vi "UpdateOverlay.vi"(7 "ROI Entry":T9 {"Analysis_Setting"."Analysis_Type" items=["None", "PatternMatch", "Edge Detection", "Barcode 1D", "Barcode 2D", "Clamp", "Clamp MAX", "Particle", "Histogram", "Straight Edge", "Circle", "Shape Detect", "OCR", "Contour", "ColorMatch"]}, 8 "error in (no error)":errorcluster, 10 "AnalysisResult":variant) -> (0 "error out":errorcluster)   [LabVIEW 2019]
uses:
  [Global] Image.vi
  [Global] Analyze Image.vi
  Analysis/Controls/Analysis_Type.ctl
  Process/Controls/Process_Type.ctl
  Process/Controls/Process_Setting.ctl
  Analysis/Controls/Analysis_Setting.ctl
  Controls/Vision_DataEntry.ctl
  <vilib>/vision/Measure.llb/Edge New.ctl
panel:
  in  "Straight Edge Cluster Array":T1(array[cluster])
  in  "Clamp output cluster":T2
  in  "Particle output cluster":T3
  in  "Clamp MAX output cluster":T4
  in  "Barcode 1D output cluster":T5
  in  "Edge Detectionoutput cluster":T7 {"?"."Edge Information"."Distance (Real-World)" format="%.2f"; "?"."Edge Information"."Location (Real-World)"."Y" format="%.2g"; "?"."Edge Information"."Location (Real-World)"."X" format="%.2f"; "?"."Edge Information"."Noise" format="%.2f"; "?"."Edge Information"."Location (Pixel)"."Y" format="%.2g"; "?"."Edge Information"."Location (Pixel)"."X" format="%.2f"; "?"."Edge Information"."Strength" format="%.2f"; "?"."Edge Information"."Distance (Pixel)" format="%.2f"}
  in  "Barcode 2D output cluster":T8
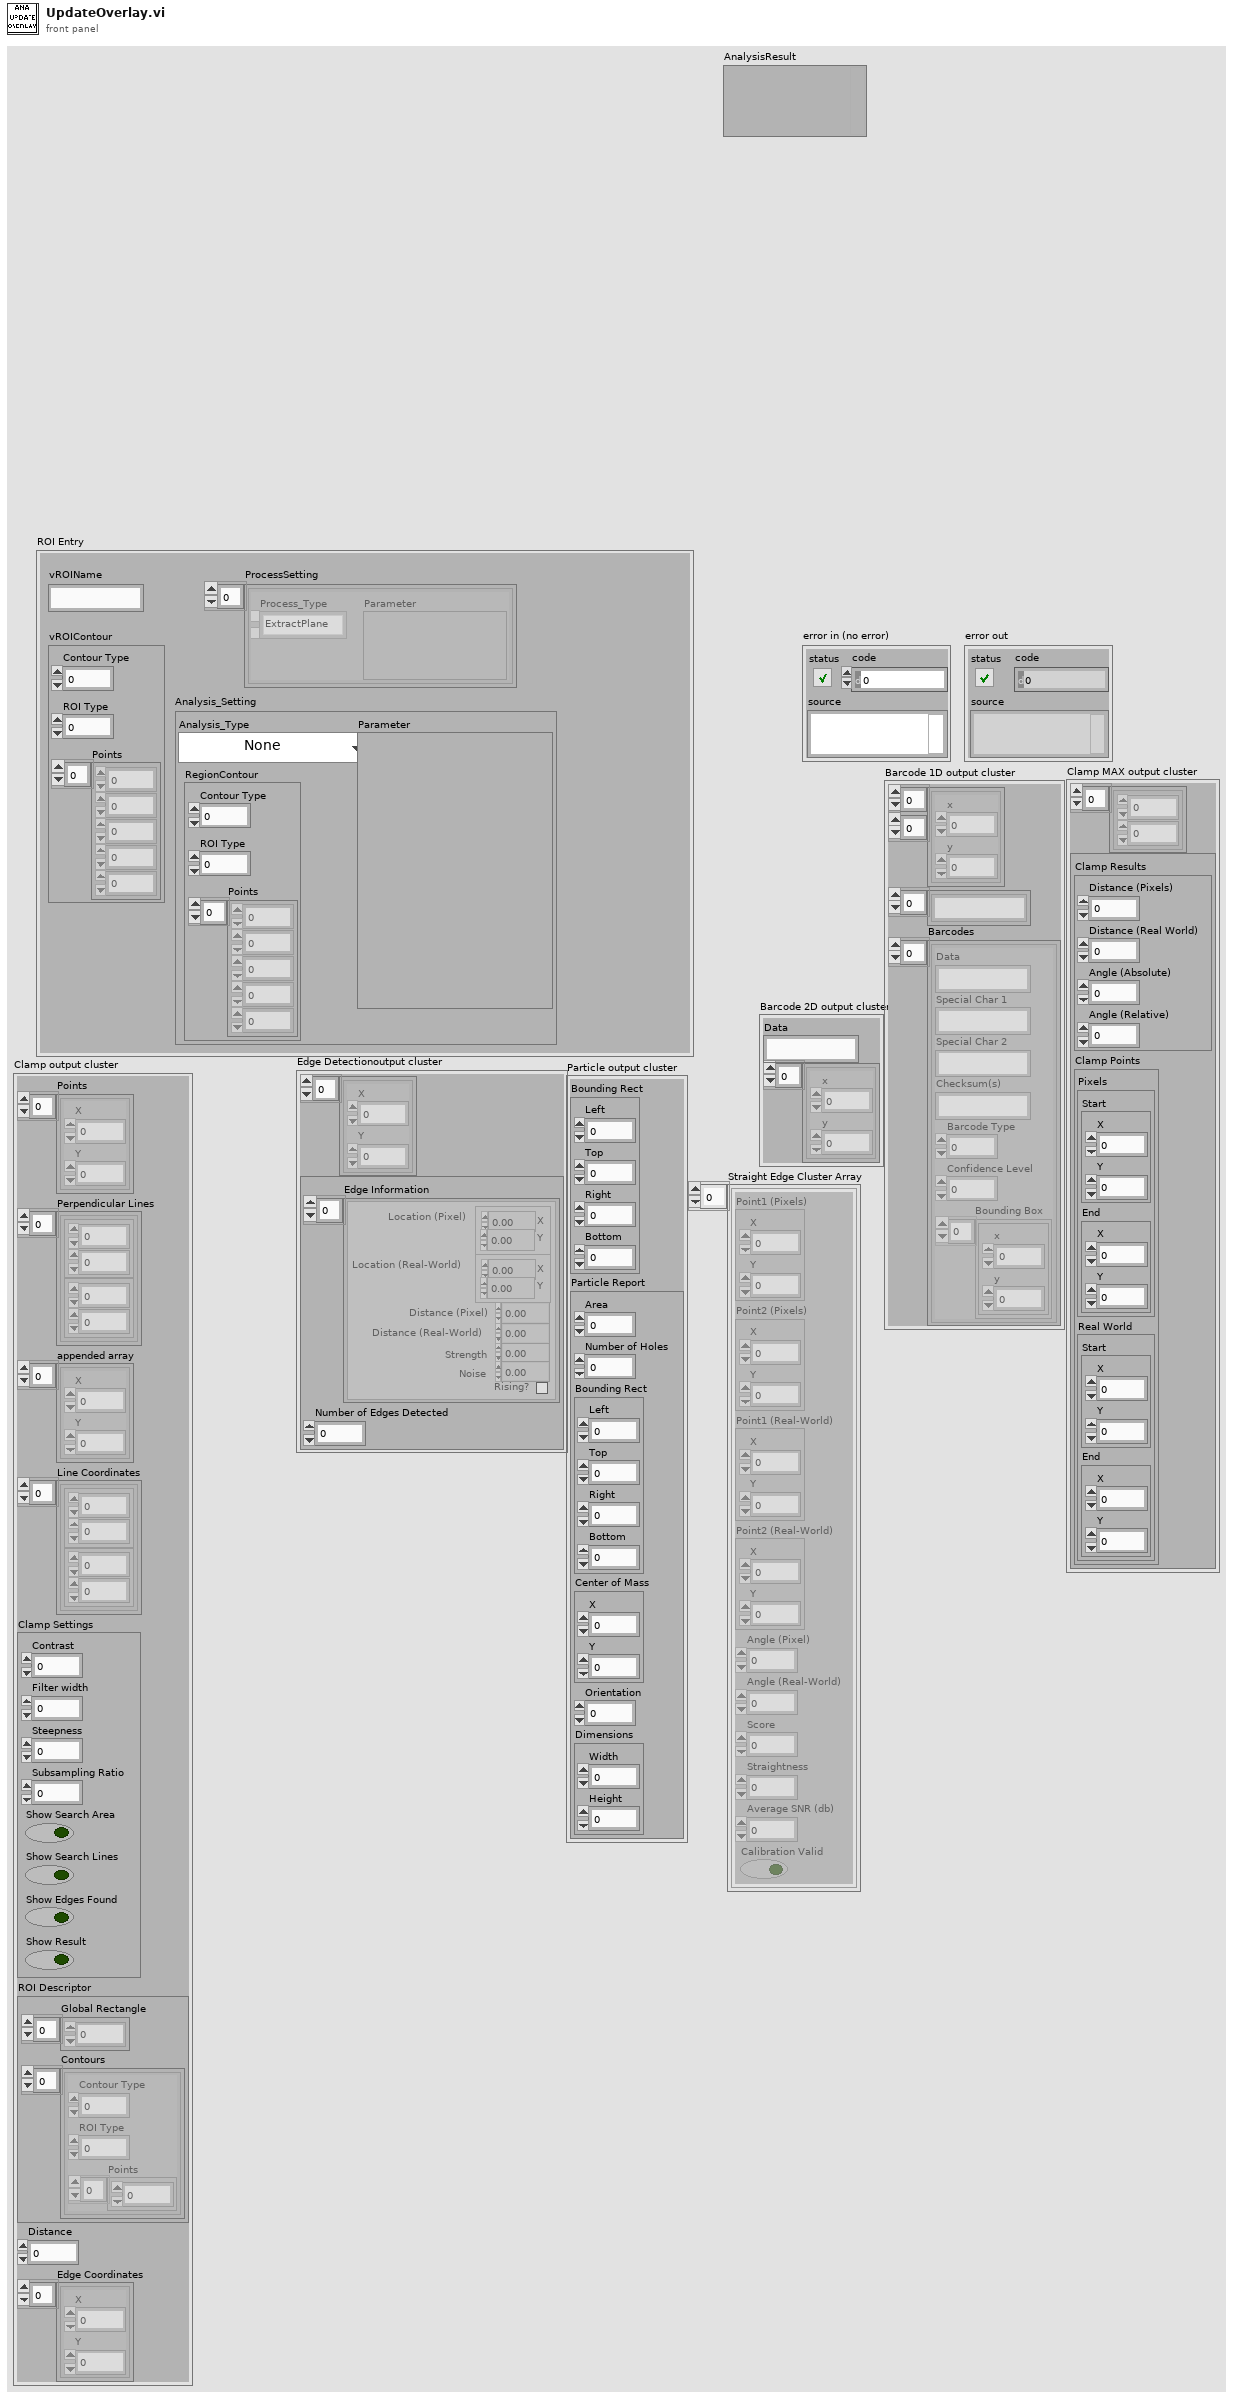
[diagram p1: front panel]
types:
  T1 = cluster{"Point1 (Pixels)":cluster{"X":sgl, "Y":sgl}, "Point2 (Pixels)":cluster{"X":sgl, "Y":sgl}, "Point1 (Real-World)":cluster{"X":sgl, "Y":sgl}, "Point2 (Real-World)":cluster{"X":sgl, "Y":sgl}, "Angle (Pixel)":dbl, "Angle (Real-World)":dbl, "Score":dbl, "Straightness":dbl, "Average SNR (db)":dbl, "Calibration Valid":bool}[]
  T2 = cluster{"Points":cluster{"X":sgl, "Y":sgl}[], "Perpendicular Lines":cluster{cluster{sgl, sgl}, cluster{sgl, sgl}}[], "appended array":cluster{"X":sgl, "Y":sgl}[], "Line Coordinates":cluster{cluster{sgl, sgl}, cluster{sgl, sgl}}[], "Clamp Settings":cluster{"Contrast":i32, "Filter width":i32, "Steepness":i32, "Subsampling Ratio":u32, "Show Search Area":bool, "Show Search Lines":bool, "Show Edges Found":bool, "Show Result":bool}, "ROI Descriptor":cluster{"Global Rectangle":i32[], "Contours":cluster{"Contour Type":u32, "ROI Type":u32, "Points":i32[]}[]}, "Distance":sgl, "Edge Coordinates":cluster{"X":sgl, "Y":sgl}[]}
  T3 = cluster{"Bounding Rect":cluster{"Left":dbl, "Top":dbl, "Right":dbl, "Bottom":dbl}, "Particle Report":cluster{"Area":dbl, "Number of Holes":dbl, "Bounding Rect":cluster{"Left":dbl, "Top":dbl, "Right":dbl, "Bottom":dbl}, "Center of Mass":cluster{"X":dbl, "Y":dbl}, "Orientation":dbl, "Dimensions":cluster{"Width":dbl, "Height":dbl}}}
  T4 = cluster{cluster{dbl, dbl}[], cluster{"Clamp Results":cluster{"Distance (Pixels)":dbl, "Distance (Real World)":dbl, "Angle (Absolute)":dbl, "Angle (Relative)":dbl}, "Clamp Points":cluster{"Pixels ":cluster{"Start":cluster{"X":dbl, "Y":dbl}, "End":cluster{"X":dbl, "Y":dbl}}, "Real World":cluster{"Start":cluster{"X":dbl, "Y":dbl}, "End":cluster{"X":dbl, "Y":dbl}}}}}
  T5 = cluster{cluster{"x":sgl, "y":sgl}[][], string[], "Barcodes":cluster{"Data":string, "Special Char 1":string, "Special Char 2":string, "Checksum(s)":string, "Barcode Type":u32, "Confidence Level":sgl, "Bounding Box":cluster{"x":sgl, "y":sgl}[]}[]}
  T6 = typedef "Edge New.ctl" = cluster{"Location (Pixel)":cluster{"X":sgl, "Y":sgl}, "Location (Real-World)":cluster{"X":sgl, "Y":sgl}, "Distance (Pixel)":dbl, "Distance (Real-World)":dbl, "Strength":dbl, "Noise":dbl, "Rising?":bool}
  T7 = cluster{cluster{"X":sgl, "Y":sgl}[], cluster{"Edge Information":T6[], "Number of Edges Detected":i32}}
  T8 = cluster{"Data":string, cluster{"x":sgl, "y":sgl}[]}
  T9 = typedef "Vision_DataEntry.ctl" = cluster{"vROIName":string, "vROIContour":cluster{"Contour Type":u32, "ROI Type":u32, "Points":i32[]}, "ProcessSetting":T10[], "Analysis_Setting":T12}
  T10 = typedef "Process_Setting.ctl" = cluster{"Process_Type":T11, "Parameter":variant}
  T11 = typedef "Process_Type.ctl" = enum16{"None", "ExtractPlane", "BinaryMono", "Operators", "GrayMorphology", "Filters", "Lookup Table", "Particle Filter", "Mask"}
  T12 = typedef "Analysis_Setting.ctl" = cluster{"Analysis_Type":T13, "RegionContour":cluster{"Contour Type":u32, "ROI Type":u32, "Points":i32[]}, "Parameter":variant}
  T13 = typedef "Analysis_Type.ctl" = u16
  T14 = typedef "IMAQ Image.ctl" = refnum<image>
  T15 = typedef "ROI Descriptor" = cluster{"Global Rectangle":i32[], "Contours":cluster{"ID":enum32{"External", "Internal"}, "Type":u32, "Coordinates":i32[]}[]}
  T16 = cluster{"ROI Descriptor out":T15, cluster{sgl, sgl}, "Angle":sgl, "Score":sgl}[]
  T17 = typedef "IMAQ Rectangle" = cluster{"Left":i32, "Top":i32, "Right":i32, "Bottom":i32, "Rotation":dbl}
  T18 = typedef "IMAQ Point" = cluster{"X":sgl, "Y":sgl}
  T19 = cluster{"Contrast":i32, "Filter width":i32, "Steepness":i32, "Subsampling Ratio":u32, "Show Search Area":bool, "Show Search Lines":bool, "Show Edges Found":bool, "Show Result":bool}
  T20 = cluster{"Global Rectangle":i32[], "Contours":cluster{"Contour Type":u32, "ROI Type":u32, "Points":i32[]}[]}
  T21 = cluster{"Left":dbl, "Top":dbl, "Right":dbl, "Bottom":dbl}
  T22 = cluster{"ROI Descriptor out":cluster{"Global Rectangle":i32[], "Contours":cluster{"ID":enum32{"External", "Internal"}, "Type":u32, "Coordinates":i32[]}[]}, "Output value":dbl}
  T23 = cluster{"Global Rectangle":i32[], "Contours":cluster{"ID":enum32{"External", "Internal"}, "Type":u32, "Coordinates":i32[]}[]}
  T24 = cluster{"ID":enum32{"External", "Internal"}, "Type":u32, "Coordinates":i32[]}[]
  T25 = cluster{"ID":enum32{"External", "Internal"}, "Type":u32, "Coordinates":i32[]}
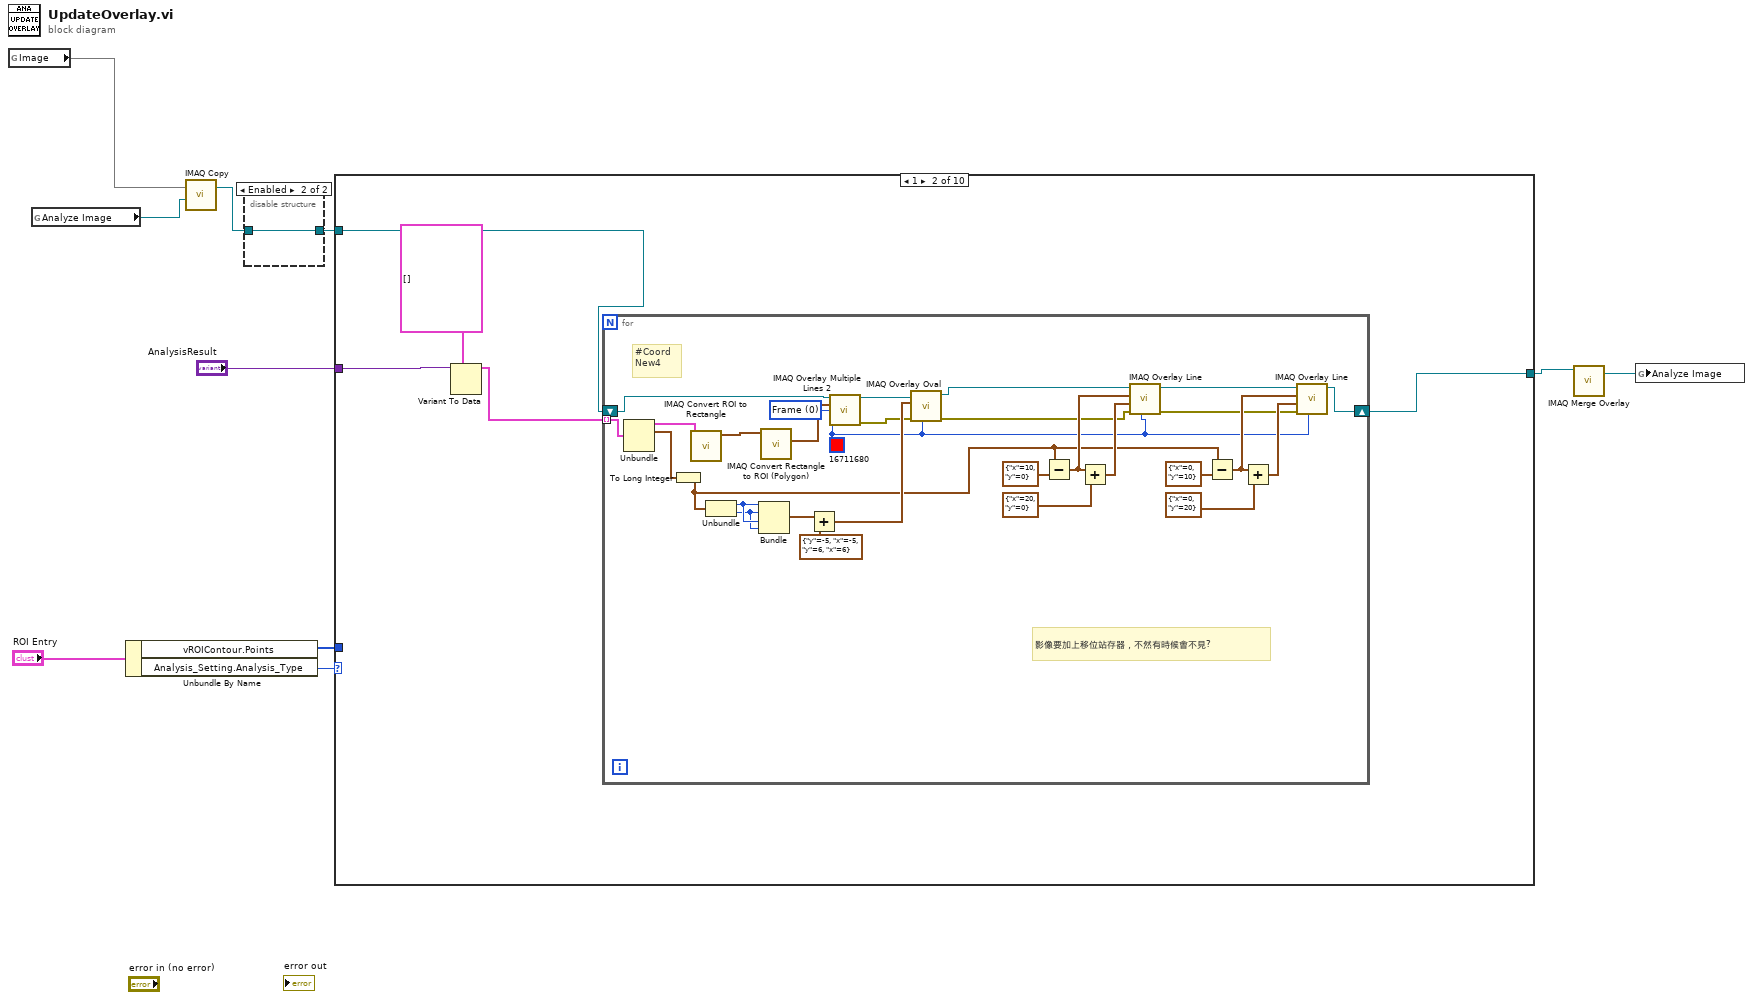
[diagram p0: block diagram]
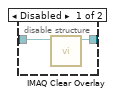
[diagram p2: hidden frame]
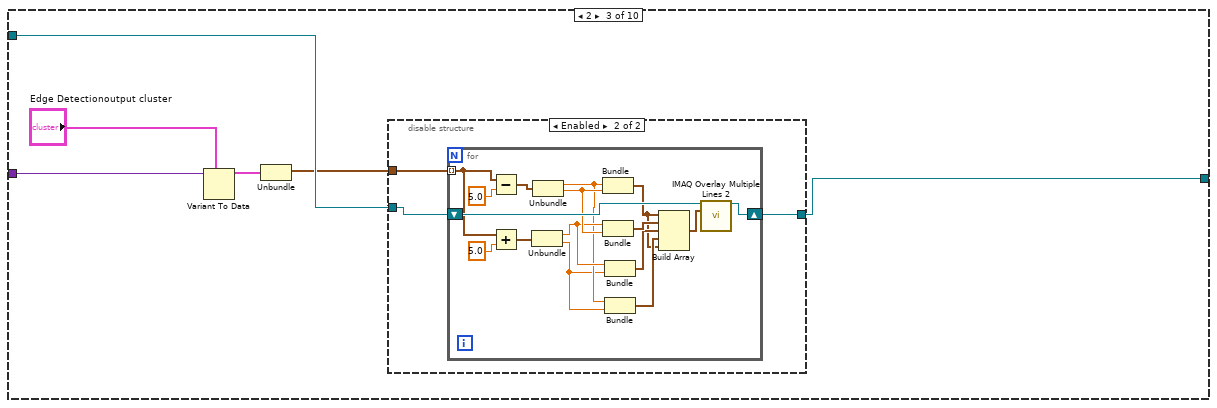
[diagram p4: hidden frame]
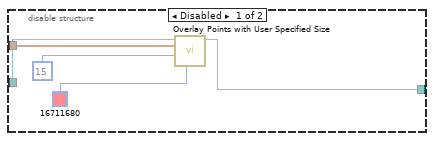
[diagram p5: hidden frame]
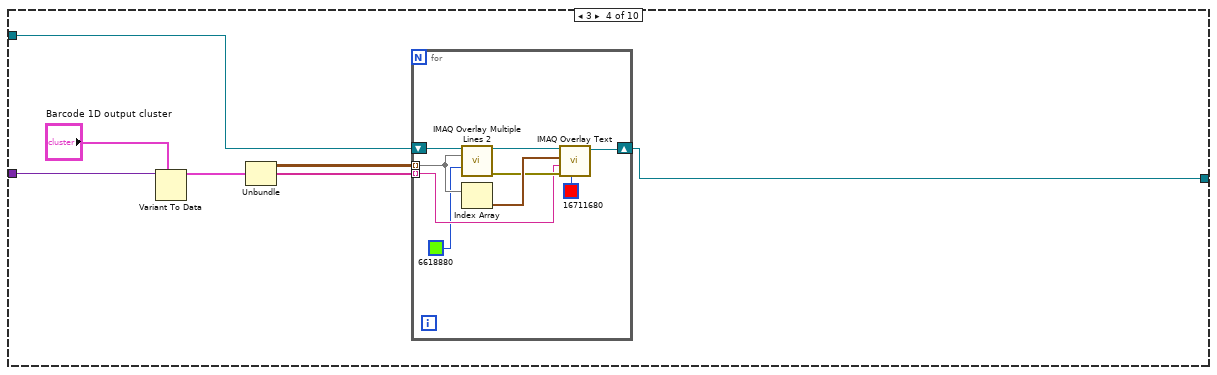
[diagram p6: hidden frame]
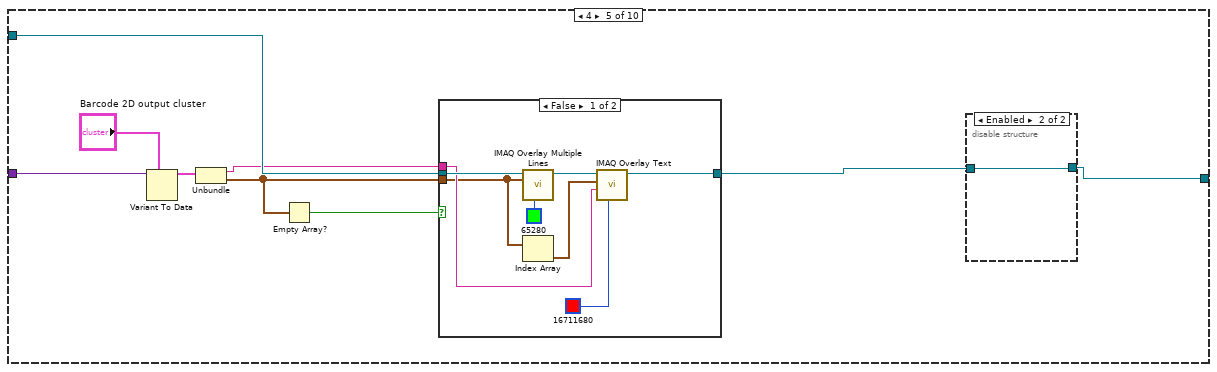
[diagram p7: hidden frame]
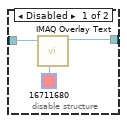
[diagram p9: hidden frame]
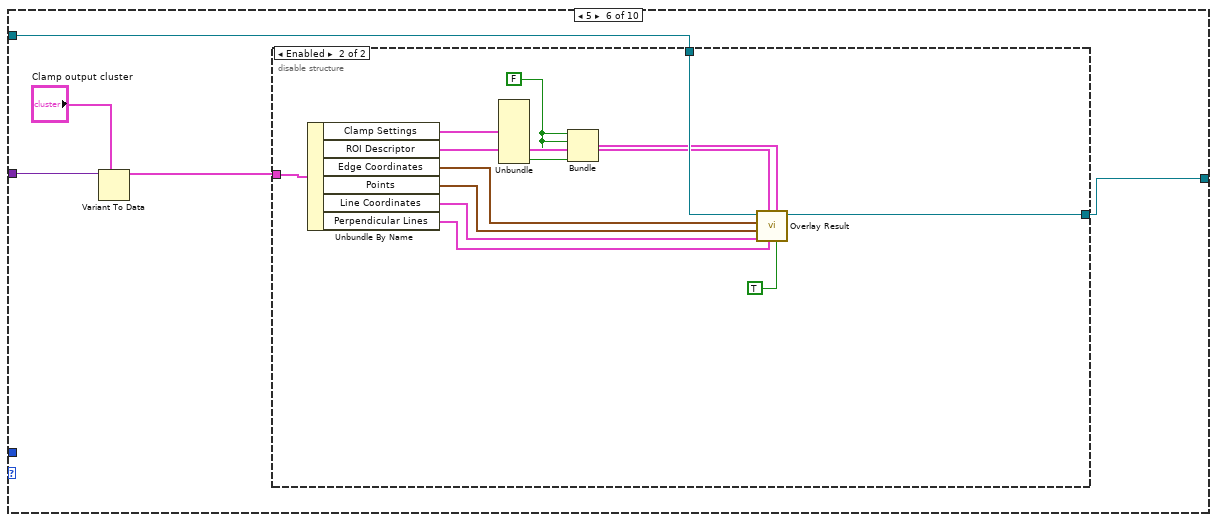
[diagram p10: hidden frame]
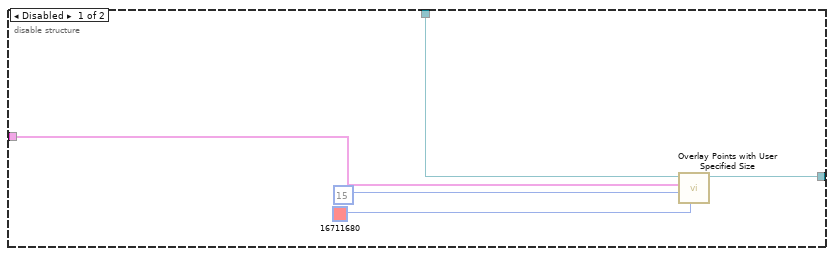
[diagram p11: hidden frame]
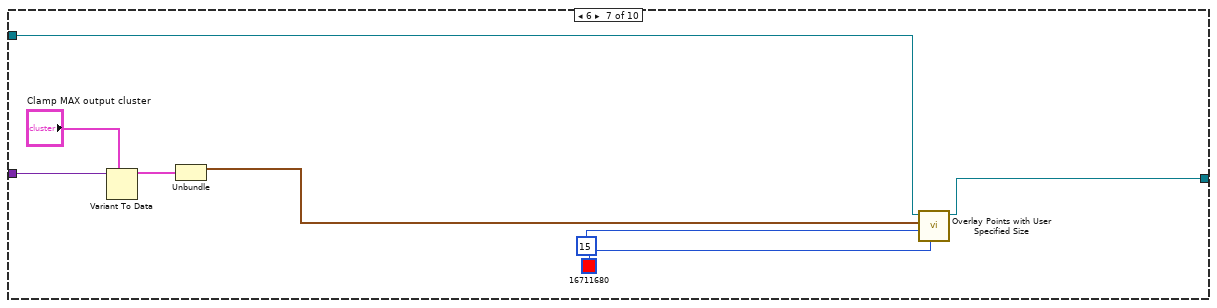
[diagram p12: hidden frame]
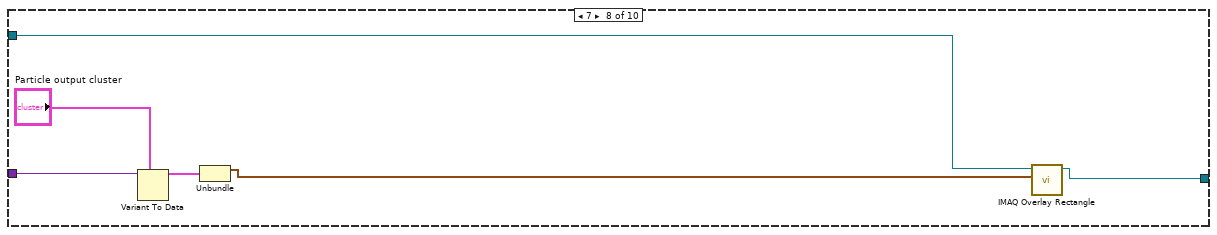
[diagram p13: hidden frame]
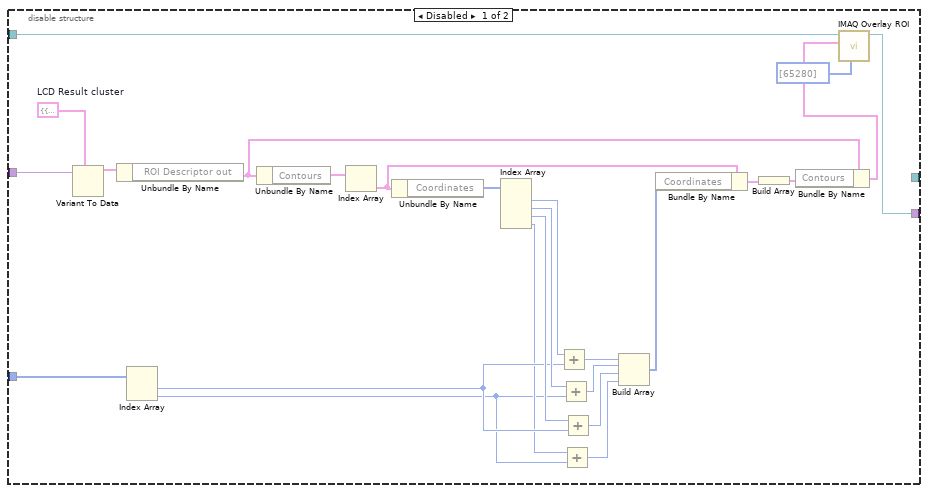
[diagram p15: hidden frame]
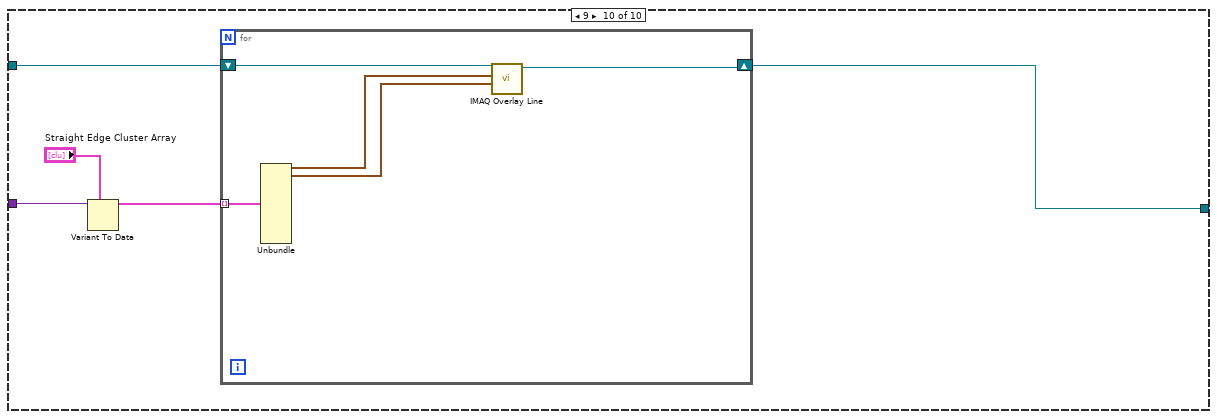
[diagram p16: hidden frame]
diagram:
  n1 = global read "[Global] Image.vi" "Image"() -> (w5)
  n2 = global read "[Global] Analyze Image.vi" "Analyze Image"() -> (w4:T14)
  n3 = Unbundle By Name("ROI Entry") -> ("vROIContour.Points"=w8:i32[], "Analysis_Setting.Analysis_Type"=w7:T13)
  n4 = call "IMAQ Copy"("Image Dst"=w4, "Image Src"=w5) -> ("Image Dst Out"=w3:T14)  [unwired: 4 in, 1 out]
  n5 = disable-structure shown="Enabled" {
    disable-tunnel: w3 -> [w12 w13]
    disable-tunnel: [w11 w13] -> w10
    frame Disabled {
      n6 = call "IMAQ Clear Overlay"("Image"=w12) -> ("Image Out"=w11:T14)  [unwired: 9 in, 1 out]
    }
    frame Enabled {
    }
  }
  n7 = case shown="1" w7 {
    tunnel: "AnalysisResult" -> [_ w19 w54 w85 w103 w121 w147 w153 w157 w189]
    tunnel: w8 -> [_ _ _ _ _ _ _ _ w155 _]
    tunnel: w10 -> [w14 w18 w53 w81 w100 w120 w144 w152 w156 w186]
    tunnel: [w14 w15 w49 w79 w95 w117 w140 w148 w154 w185] -> w1
    frame 0, Default {
    }
    frame 1 {
      n8 = Variant To Data(type=T16 [], Variant=w19) -> (data=w17:T16)  [unwired: 1 in, 1 out]
      n9 = for {
        tunnel: w17 -> [w44] mode=indexing
        shift-right: [w22] -> w15
        shift-left: w18 -> [w48]
        w45 = u32 0 items=["Frame", "Fill"] ("Drawing Mode (Frame)")
        w21 = u32 16711680 ("Color")
        # "#Coord\nNew4"
        # "影像要加上移位站存器，不然有時候會不見?"
        n10 = Unbundle(w44) -> ("ROI Descriptor out"=w43:T15, w20:cluster{sgl, sgl})  [unwired: 2 out]
        n11 = To Long Integer(number=w20) -> (32bit integer=w26:cluster{i32, i32})
        n12 = call "IMAQ Convert ROI to Rectangle"("ROI Descriptor"=w43) -> ("Rectangle"=w46:T17)  [unwired: 8 in, 1 out]
        n13 = Unbundle(w26) -> (w41:i32, w40:i32)
        n14 = Bundle(w41, w40, w41, w40) -> (w39:cluster{i32, i32, i32, i32})  [unwired: 1 out]
        n15 = call "IMAQ Convert Rectangle to ROI (Polygon)"("Rectangle"=w46) -> ("Rectangle Points"=w47:T18[])  [unwired: 7 in, 2 out]
        n16 = Add(x=w39, y=cluster{"y":i32, "x":i32, "y":i32, "x":i32} {"y"=-5, "x"=-5, "y"=6, "x"=6}) -> (x+y=w37:cluster{i32, i32, i32, i32})
        n17 = call "IMAQ Overlay Multiple Lines 2"("Image"=w48, "Line End Points"=w47, "Drawing Mode (Frame)"=w45, "Color"=w21) -> ("Image Out"=w42:T14, "error out"=w25:errorcluster)  [unwired: 10 in]
        n18 = call "IMAQ Overlay Oval"("Color"=w21, "error in (no error)"=w25, "Bounding Rectangle"=w37, "Image"=w42) -> ("error out"=w24:errorcluster, "Image Out"=w23:T14)  [unwired: 6 in]
        n19 = Subtract(x=w26, y=cluster{"x":i32, "y":i32} {"x"=10, "y"=0}) -> (x-y=w35:cluster{i32, i32})
        n20 = Add(x=w35, y=cluster{"x":i32, "y":i32} {"x"=20, "y"=0}) -> (x+y=w33:cluster{i32, i32})
        n21 = call "IMAQ Overlay Line"("Color"=w21, "error in (no error)"=w24, "End Point"=w33, "Start Point"=w35, "Image"=w23) -> ("error out"=w27:errorcluster, "Image Out"=w28:T14)  [unwired: 1 in, 4 out]
        n22 = Subtract(x=w26, y=cluster{"x":i32, "y":i32} {"x"=0, "y"=10}) -> (x-y=w31:cluster{i32, i32})
        n23 = Add(x=w31, y=cluster{"x":i32, "y":i32} {"x"=0, "y"=20}) -> (x+y=w32:cluster{i32, i32})
        n24 = call "IMAQ Overlay Line"("Color"=w21, "error in (no error)"=w27, "End Point"=w32, "Start Point"=w31, "Image"=w28) -> ("Image Out"=w22:T14)  [unwired: 1 in, 5 out]
      }
    }
    frame 2 {
      n25 = Variant To Data(type="Edge Detectionoutput cluster", Variant=w54) -> (data=w51:T7)  [unwired: 1 in, 1 out]
      n26 = Unbundle(w51) -> (w50:cluster{"X":sgl, "Y":sgl}[])  [unwired: 1 out]
      n27 = disable-structure shown="Enabled" {
        disable-tunnel: w53 -> [w59 w61]
        disable-tunnel: [w57 w60] -> w49
        disable-tunnel: w50 -> [w55 w62]
        frame Disabled {
          n28 = call "Overlay Points with User Specified Size.vi"("Color"=u32 16711680, "Point Diameter (5)"=u32 15, "Points"=w55, "Image In"=w59) -> ("Image Out"=w57:T14)  [unwired: 6 in, 1 out]
        }
        frame Enabled {
          n29 = for {
            tunnel: w62 -> [w75] mode=indexing
            shift-right: [w63] -> w60
            shift-left: w61 -> [w78]
            n30 = Subtract(x=w75, y=5.0) -> (x-y=w74:cluster{"X":dbl, "Y":dbl})
            n31 = Add(x=w75, y=5.0) -> (x+y=w73:cluster{"X":dbl, "Y":dbl})
            n32 = Unbundle(w73) -> ("X"=w71:dbl, "Y"=w69:dbl)
            n33 = Unbundle(w74) -> ("X"=w70:dbl, "Y"=w72:dbl)
            n34 = Bundle("X"=w70, "Y"=w72) -> (w65:cluster{"X":dbl, "Y":dbl})  [unwired: 1 in]
            n35 = Bundle("X"=w71, "Y"=w72) -> (w68:cluster{"X":dbl, "Y":dbl})  [unwired: 1 in]
            n36 = Bundle("X"=w71, "Y"=w69) -> (w67:cluster{"X":dbl, "Y":dbl})  [unwired: 1 in]
            n37 = Bundle("X"=w70, "Y"=w69) -> (w66:cluster{"X":dbl, "Y":dbl})  [unwired: 1 in]
            n38 = Build Array(w65, w68, w67, w66, w65) -> (w64:cluster{"X":dbl, "Y":dbl}[])
            n39 = call "IMAQ Overlay Multiple Lines 2"("Image"=w78, "Line End Points"=w64) -> ("Image Out"=w63:T14)  [unwired: 12 in, 1 out]
          }
        }
      }
    }
    frame 3 {
      n40 = Variant To Data(type="Barcode 1D output cluster", Variant=w85) -> (data=w83:T5)  [unwired: 1 in, 1 out]
      n41 = Unbundle(w83) -> (w82:cluster{"x":sgl, "y":sgl}[][], w80:string[])  [unwired: 1 out]
      n42 = for {
        tunnel: w82 -> [w89] mode=indexing
        shift-right: [w87] -> w79
        shift-left: w81 -> [w90]
        tunnel: w80 -> [w88] mode=indexing
        n43 = call "IMAQ Overlay Multiple Lines 2"("Image"=w90, "Line End Points"=w89, "Color"=u32 6618880) -> ("Image Out"=w91:T14, "error out"=w93:errorcluster)  [unwired: 11 in]
        n44 = Index Array(array=w89) -> (element=w94:cluster{"x":sgl, "y":sgl})  [unwired: 1 in]
        n45 = call "IMAQ Overlay Text"("Text Color (black)"=u32 16711680, "error in (no error)"=w93, "String"=w88, "Origin"=w94, "Image"=w91) -> ("Image Out"=w87:T14)  [unwired: 5 in, 1 out]
      }
    }
    frame 4 {
      n46 = Variant To Data(type="Barcode 2D output cluster", Variant=w103) -> (data=w101:T8)  [unwired: 1 in, 1 out]
      n47 = Unbundle(w101) -> ("Data"=w96:string, w98:cluster{"x":sgl, "y":sgl}[])
      n48 = Empty Array?(array=w98) -> (empty?=w97:bool)
      n49 = case shown="False" w97 {
        tunnel: w100 -> [w110 w112]
        tunnel: [w108 w112] -> w99
        tunnel: w98 -> [w106 _]
        tunnel: w96 -> [w107 _]
        frame False {
          n50 = call "IMAQ Overlay Multiple Lines"("Color"=u32 65280, "Line End Points"=w106, "Image"=w110) -> ("Image Out"=w109:T14)  [unwired: 7 in, 1 out]
          n51 = Index Array(array=w106) -> (element=w105:cluster{"x":sgl, "y":sgl})  [unwired: 1 in]
          n52 = call "IMAQ Overlay Text"("Text Color (black)"=u32 16711680, "String"=w107, "Origin"=w105, "Image"=w109) -> ("Image Out"=w108:T14)  [unwired: 6 in, 1 out]
        }
        frame True {
        }
      }
      n53 = disable-structure shown="Enabled" {
        disable-tunnel: w99 -> [w114 w116]
        disable-tunnel: [w113 w116] -> w95
        frame Disabled {
          n54 = call "IMAQ Overlay Text"("Text Color (black)"=u32 16711680, "Image"=w114) -> ("Image Out"=w113:T14)  [unwired: 8 in, 1 out]
        }
        frame Enabled {
        }
      }
    }
    frame 5 {
      n55 = Variant To Data(type="Clamp output cluster", Variant=w121) -> (data=w118:T2)  [unwired: 1 in, 1 out]
      n56 = disable-structure shown="Enabled" {
        disable-tunnel: w120 -> [w124 w139]
        disable-tunnel: [w123 w138] -> w117
        disable-tunnel: w118 -> [w122 w127]
        frame Disabled {
          n57 = call "Overlay Points with User Specified Size.vi"("Color"=u32 16711680, "Point Diameter (5)"=u32 15, "Points"=w122, "Image In"=w124) -> ("Image Out"=w123:T14)  [unwired: 6 in, 1 out]
        }
        frame Enabled {
          w129 = FALSE
          n58 = Unbundle By Name(w127) -> ("Clamp Settings"=w132:T19, "ROI Descriptor"=w133:T20, "Edge Coordinates"=w130:cluster{"X":sgl, "Y":sgl}[], "Points"=w134:cluster{"X":sgl, "Y":sgl}[], "Line Coordinates"=w135:cluster{cluster{sgl, sgl}, cluster{sgl, sgl}}[], "Perpendicular Lines"=w136:cluster{cluster{sgl, sgl}, cluster{sgl, sgl}}[])
          n59 = Unbundle(w132) -> ("Show Result"=w128:bool)  [unwired: 7 out]
          n60 = Bundle(w129, w129, w129, "Show Result"=w128) -> (w131:cluster{bool, bool, bool, "Show Result":bool})  [unwired: 1 in]
          n61 = call "Overlay Result.vi"("Min / Max"=TRUE, "Setup"=w131, "Perpendicular Lines"=w136, "ROI Descriptor"=w133, "Search Lines"=w135, "All Edges Found"=w134, "Measurement Edges"=w130, "Image In"=w139) -> ("Image Out"=w138:T14)  [unwired: 3 in]
        }
      }
    }
    frame 6 {
      n62 = Variant To Data(type="Clamp MAX output cluster", Variant=w147) -> (data=w142:T4)  [unwired: 1 in, 1 out]
      n63 = Unbundle(w142) -> (w141:cluster{dbl, dbl}[])  [unwired: 1 out]
      n64 = call "Overlay Points with User Specified Size.vi"("Color"=u32 16711680, "Point Diameter (5)"=u32 15, "Points"=w141, "Image In"=w144) -> ("Image Out"=w140:T14)  [unwired: 6 in, 1 out]
    }
    frame 7 {
      n65 = Variant To Data(type="Particle output cluster", Variant=w153) -> (data=w150:T3)  [unwired: 1 in, 1 out]
      n66 = Unbundle(w150) -> ("Bounding Rect"=w149:T21)  [unwired: 1 out]
      n67 = call "IMAQ Overlay Rectangle"("Rectangle"=w149, "Image"=w152) -> ("Image Out"=w148:T14)  [unwired: 8 in, 1 out]
    }
    frame 8 {
      n68 = disable-structure shown="Enabled" {
        disable-tunnel: w157 -> [w182 w184]
        disable-tunnel: w156 -> [w180 w183]
        disable-tunnel: [w178 w184] -> _
        disable-tunnel: w155 -> [w177 _]
        disable-tunnel: [_ w183] -> w154
        frame Disabled {
          w181 = T22 {"ROI Descriptor out"={"Global Rectangle"=[], "Contours"=[]}, "Output value"=0.0}  # LCD Result cluster
          n69 = Variant To Data(type=w181, Variant=w182) -> (data=w160:T22)  [unwired: 1 in, 1 out]
          n70 = Unbundle By Name(w160) -> ("ROI Descriptor out"=w159:T23)
          n71 = Index Array(array=w177) -> (element #1=w171:i32, element #2=w169:i32)  [unwired: 2 in]
          n72 = Unbundle By Name(w159) -> ("Contours"=w176:T24)
          n73 = Index Array(array=w176) -> (element=w164:T25)  [unwired: 1 in]
          n74 = Unbundle By Name(w164) -> ("Coordinates"=w175:i32[])
          n75 = Index Array(array=w175) -> (element #1=w174:i32, element #2=w173:i32, element #3=w172:i32, element #4=w170:i32)  [unwired: 4 in]
          n76 = Add(x=w174, y=w171) -> (x+y=w168:i32)
          n77 = Add(x=w173, y=w169) -> (x+y=w167:i32)
          n78 = Add(x=w170, y=w169) -> (x+y=w165:i32)
          n79 = Add(x=w172, y=w171) -> (x+y=w166:i32)
          n80 = Build Array(w168, w167, w166, w165) -> (w163:i32[])
          n81 = Bundle By Name(cluster=w164, "Coordinates"=w163) -> (w162:T25)
          n82 = Build Array(w162) -> (w161:T24)
          n83 = Bundle By Name(cluster=w159, "Contours"=w161) -> (w158:T23)
          n84 = call "IMAQ Overlay ROI"("Colors (Green)"=u32[] [65280], "ROI Descriptor"=w158, "Image"=w180) -> ("Image Out"=w178:T14)  [unwired: 7 in, 1 out]
        }
        frame Enabled {
        }
      }
    }
    frame 9 {
      n85 = Variant To Data(type="Straight Edge Cluster Array", Variant=w189) -> (data=w188:T1)  [unwired: 1 in, 1 out]
      n86 = for {
        tunnel: w188 -> [w194] mode=indexing
        shift-right: [w192] -> w185
        shift-left: w186 -> [w193]
        n87 = Unbundle(w194) -> ("Point1 (Pixels)"=w191:cluster{"X":sgl, "Y":sgl}, "Point2 (Pixels)"=w190:cluster{"X":sgl, "Y":sgl})  [unwired: 8 out]
        n88 = call "IMAQ Overlay Line"("End Point"=w190, "Start Point"=w191, "Image"=w193) -> ("Image Out"=w192:T14)  [unwired: 7 in, 1 out]
      }
    }
  }
  n89 = call "IMAQ Merge Overlay"("Image Src"=w1) -> ("Image Dst Out"=w2:T14)  [unwired: 9 in, 1 out]
  n90 = global write "[Global] Analyze Image.vi" "Analyze Image"(w2) -> ()
